vi "NearestDistanceGlobal.vi"() -> ()   [LabVIEW 2016]
panel:
  out "nearest distance":dbl
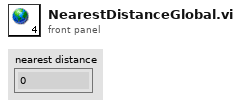
[diagram p1: front panel]
diagram:
